vi "FTW-Container-Name-Get.vi"(8 "error in (no error)":errorcluster, 11 "FTW-Container in":refnum<class "FTW-Container.lvclass">) -> (0 "error out":errorcluster, 2 "Name":string, 3 "FTW-Container out":refnum<class "FTW-Container.lvclass">)   [LabVIEW 2015, in "FTW-Container.lvclass"]
uses:
  FTW-Container.lvclass
  FTW-Container.lvclass/FTW-Container.ctl
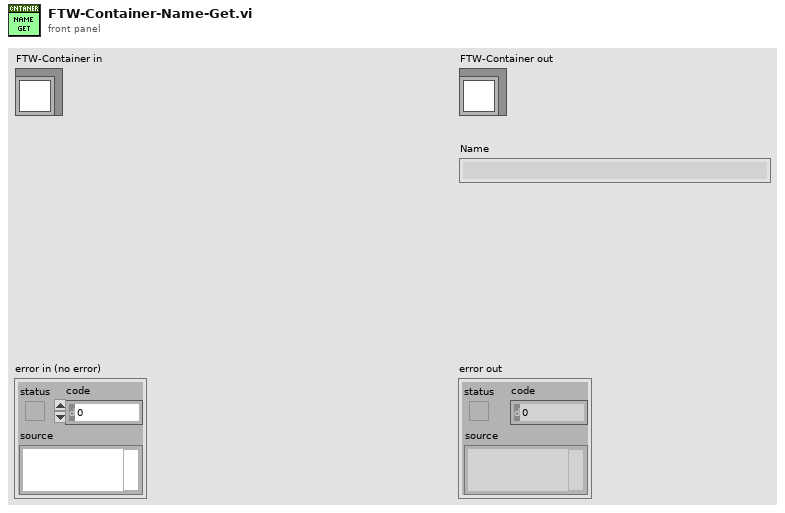
[diagram p1: front panel]
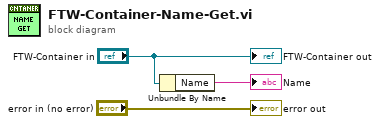
[diagram p0: block diagram]
diagram:
  n1 = Unbundle By Name("FTW-Container in") -> ("Name"=→"Name":string)
  "error out" <- "error in (no error)"
  "FTW-Container out" <- "FTW-Container in"
